vi "SR7265 Read DAQs.vi"(8 "Error In":errorcluster, 11 "VISA resource":refnum<visa-resource-name>) -> (0 "Error Out":errorcluster, 2 "Data":dbl[](array[numeric]), 3 "VISA resource dup":refnum<visa-resource-name>)   [LabVIEW 2019]
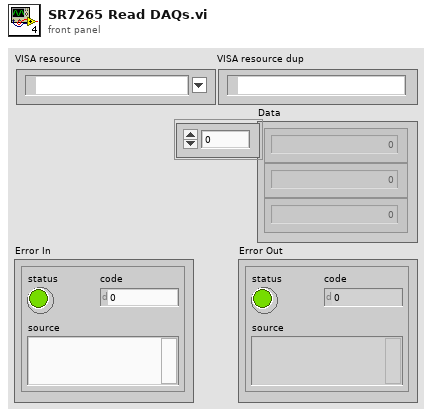
[diagram p1: front panel]
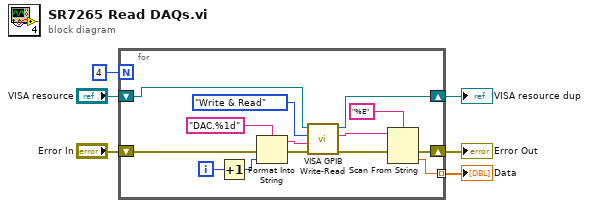
[diagram p0: block diagram]
diagram:
  n1 = for {
    N: 4 -> [_]
    shift-right: [w7] -> w1
    shift-left: "Error In" -> [w14]
    shift-right: [w13] -> w3
    shift-left: "VISA resource" -> [w12]
    tunnel: [w9] -> w2 mode=indexing
    i -> [w16]
    n2 = Increment(x=w16) -> (x+1=w15:i32)
    n3 = Format Into String(format string="DAC.%1d", error in=w14, w15) -> (resulting string=w18:string, error out=w17:errorcluster)  [unwired: 1 in]
    n4 = call "VISA GPIB Write-Read.vi"("error in (no error)"=w17, "Command"=w18, "Action"=enum16{"Write", "Read", "Write & Read"}."Write & Read", "VISA resource name"=w12) -> ("error out"=w8:errorcluster, "String Returned"=w11:string, "dup VISA Session"=w13:refnum<visa-resource-name>)  [unwired: 4 in, 1 out]
    n5 = Scan From String(format string="%E", input string=w11, error in=w8) -> (error out=w7:errorcluster, output 1=w9:dbl)  [unwired: 2 in, 2 out]
  }
  "VISA resource dup" <- w3
  "Data" <- w2
  "Error Out" <- w1
